vi "Do.vi"(8 "error in (no error)":errorcluster, 10 "Ctl Refnum in":refnum<vi>, 11 "ControlAction in":refnum<class "ControlDoBase.lvclass">) -> (0 "error out":errorcluster, 2 "Ctl Refnum out":refnum<vi>, 3 "ControlAction out":refnum<class "ControlDoBase.lvclass">)   [LabVIEW 2016, in "VI.lvlib" / "ControlDoBase.lvclass"]
uses:
  ControlDoBase.lvclass
  ControlDoBase.lvclass/ControlDoBase.ctl
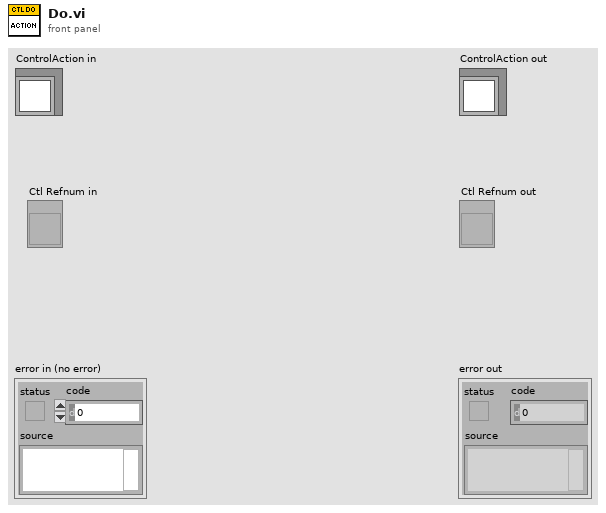
[diagram p1: front panel]
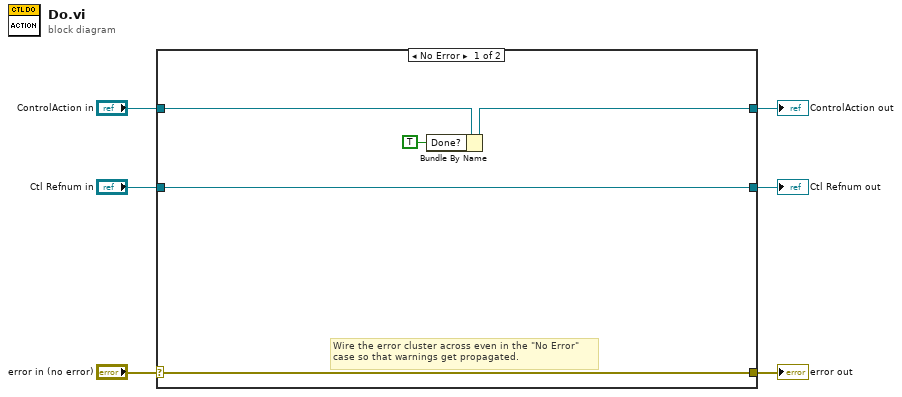
[diagram p0: block diagram]
diagram:
  n1 = case shown="No Error" "error in (no error)" {
    selector: "error in (no error)" -> [w10 w14]
    tunnel: [w10 w14] -> w5
    tunnel: [w8 w13] -> w3
    tunnel: "ControlAction in" -> [w11 w13]
    tunnel: [w9 w12] -> w2
    tunnel: "Ctl Refnum in" -> [w9 w12]
    frame No Error {
      # "Wire the error cluster across even in the \"No Error\"\ncase so that warnings get propagated."
      n2 = Bundle By Name(cluster=w11, "Done?"=TRUE) -> (w8:refnum<class "ControlDoBase.lvclass">)
    }
    frame Error {
    }
  }
  "error out" <- w5
  "ControlAction out" <- w3
  "Ctl Refnum out" <- w2
